vi "SetStatus.vi"(8 "error in (no error)":errorcluster caption="错误输入（无错误）", 10 "Status":bool, 11 "Timer 输入":refnum<class "Timer.lvclass">) -> (0 "error out":errorcluster caption="错误输出", 3 "Timer 输出":refnum<class "Timer.lvclass">)   [LabVIEW 2018, in "Timer.lvclass"]
uses:
  Timer.lvclass
  Timer.lvclass/Timer.ctl
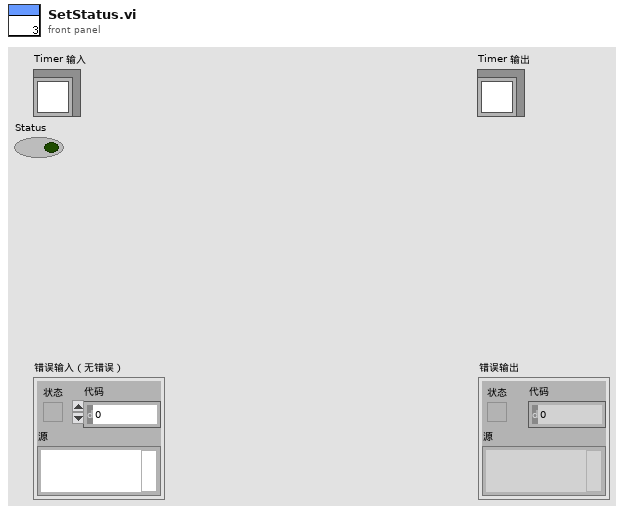
[diagram p1: front panel]
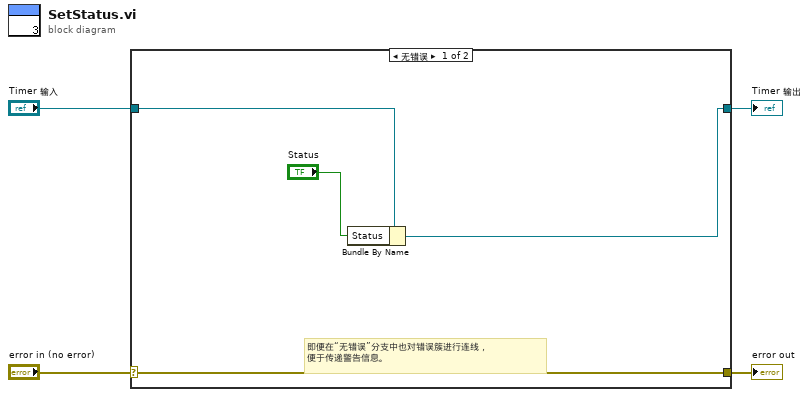
[diagram p0: block diagram]
diagram:
  n1 = case shown="无错误" "error in (no error)" {
    selector: "error in (no error)" -> [w8 w10]
    tunnel: [w8 w10] -> w3
    tunnel: [w6 w9] -> w1
    tunnel: "Timer 输入" -> [w7 w9]
    frame No Error {
      # "即便在“无错误”分支中也对错误簇进行连线，\n便于传递警告信息。"
      n2 = Bundle By Name(cluster=w7, "Status"="Status") -> (w6:refnum<class "Timer.lvclass">)
    }
    frame Error {
    }
  }
  "error out" <- w3
  "Timer 输出" <- w1
